vi "Set Printing Flow.vi"(8 "error in (no error)":errorcluster, 10 "Print Value":dbl, 11 "MFC Actor.lvlib:MFC.lvclass":refnum<class "MFC.lvclass">) -> (0 "error out":errorcluster, 3 "MFC Actor.lvlib:MFC.lvclass 2":refnum<class "MFC.lvclass">)   [LabVIEW 2018, in "MFC Actor.lvlib" / "MFC.lvclass"]
uses:
  MFC.lvclass
  MFC.lvclass/MFC.ctl
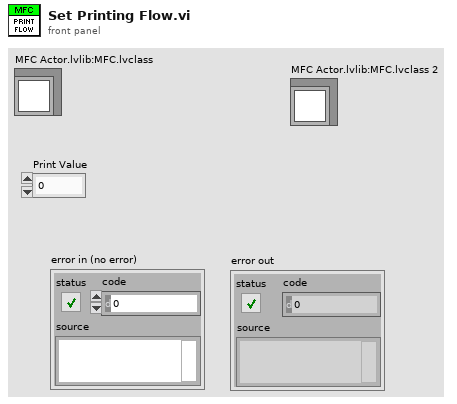
[diagram p1: front panel]
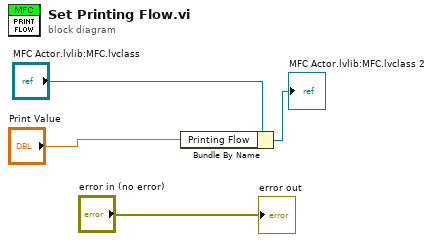
[diagram p0: block diagram]
diagram:
  n1 = Bundle By Name(cluster="MFC Actor.lvlib:MFC.lvclass", "Printing Flow"="Print Value") -> (→"MFC Actor.lvlib:MFC.lvclass 2":refnum<class "MFC.lvclass">)
  "error out" <- "error in (no error)"
